vi "诊断标定3.vi"(8 "CAN端口":u16(ring), 9 "设备索引号":u16(ring), 10 "CAN卡类型":u32(ring)=21) -> ()   [LabVIEW 2013] (continued)
          tunnel: w3642 -> [w3645 w3652]
          tunnel: [w3646 w3651] -> w3641
          tunnel: [w3645 w3650] -> w3640
          frame False {
          }
          frame True {
            n2857 = global read "EV05全局变量1.vi" "授权功能"() -> (w3648:bool)
            n2858 = case shown="假" w3648 {
              tunnel: [TRUE ("发送成功") w3672] -> w3649
              frame False {
              }
              frame True {
                n2859 = local read "设备索引号"() -> (w3667:u16)
                n2860 = local read "CAN卡类型"() -> (w3668:u32)
                n2861 = local read "CAN端口"() -> (w3666:u16)
                n2862 = call "标定授权发送.vi"("CAN卡类型"=w3668, "解锁类型"=enum16{"读取", "写", "下载"}."读取", "设备索引号"=w3667, "CAN端口"=w3666, "是否连接"=TRUE, "板选择"=0, "FUNC"=u32 0) -> ("发送成功"=w3672:bool)  [unwired: 8 out]
              }
            }
            n2863 = stacked-sequence {
              tunnel: [w3656] -> w3647
              frame #0 {
                w3656 = TRUE ("控制1")
                w3660 = FALSE ("写?")
                n2864 = call <vilib>:"Set Busy.vi"("disable click? (T)"=FALSE) -> ()  [unwired: 3 in, 8 out]
                n2865 = local write "写?"(w3660) -> ()
                n2866 = global write "EV05全局变量1.vi" "写入超时"(w3660) -> ()
                n2867 = local write "平台软件版本号"(" " ("平台软件版本号")) -> ()
                n2868 = local write "控制1"(w3656) -> ()
                n2869 = local write "消除"(TRUE ("消除")) -> ()
                n2870 = property on="保存版本信息" class="Bool (严格)"("Visible"=TRUE ("可见")) -> ()  [unwired: 2 in, 2 out]
                n2871 = global write "EV05全局变量1.vi" "流控帧 2"(TRUE ("流控帧 2")) -> ()
                n2872 = local write "主从选择"(enum32{"主板", "从板"}."主板" ("主从选择")) -> ()
                n2873 = local write "清BUFF"(FALSE ("清BUFF")) -> ()
                n2874 = global write "EV05全局变量1.vi" "流控帧"(FALSE ("流控帧")) -> ()
              }
            }
            n2875 = case shown="真" w3649 {
              tunnel: w3653 -> [w3674 w3679]
              tunnel: w3652 -> [w3673 w3678]
              tunnel: [w3674 w3676] -> w3651
              tunnel: [w3673 w3675] -> w3650
              tunnel: w3647 -> [_ _]
              frame False {
              }
              frame True {
                n2876 = Enqueue Element(queue=w3679, element="平台软件版本读取" ("元素"), error in (no error)=w3678) -> (queue out=w3676:refnum<queue>, error out=w3675:errorcluster)  [unwired: 2 out]
              }
            }
          }
        }
      }
      event "模块版本读取": Value Change {
        n2877 = event-data() -> ("NewVal"=w3684:bool)  [unwired: 5 out]
        n2878 = case shown="真" w3684 {
          tunnel: w3683 -> [w3686 w3693]
          tunnel: w3682 -> [w3685 w3692]
          tunnel: [w3686 w3691] -> w3681
          tunnel: [w3685 w3690] -> w3680
          frame False {
          }
          frame True {
            n2879 = global read "EV05全局变量1.vi" "授权功能"() -> (w3688:bool)
            n2880 = case shown="假" w3688 {
              tunnel: [TRUE ("发送成功") w3711] -> w3689
              frame False {
              }
              frame True {
                n2881 = local read "设备索引号"() -> (w3706:u16)
                n2882 = local read "CAN卡类型"() -> (w3707:u32)
                n2883 = local read "CAN端口"() -> (w3705:u16)
                n2884 = call "标定授权发送.vi"("CAN卡类型"=w3707, "解锁类型"=enum16{"读取", "写", "下载"}."读取", "设备索引号"=w3706, "CAN端口"=w3705, "是否连接"=TRUE, "板选择"=0, "FUNC"=u32 0) -> ("发送成功"=w3711:bool)  [unwired: 8 out]
              }
            }
            n2885 = stacked-sequence {
              tunnel: [w3696] -> w3687
              frame #0 {
                w3696 = TRUE ("控制1")
                w3699 = FALSE ("写?")
                n2886 = call <vilib>:"Set Busy.vi"("disable click? (T)"=FALSE) -> ()  [unwired: 3 in, 8 out]
                n2887 = local write "写?"(w3699) -> ()
                n2888 = global write "EV05全局变量1.vi" "写入超时"(w3699) -> ()
                n2889 = local write "主从选择"(enum32{"主板", "从板"}."主板" ("主从选择")) -> ()
                n2890 = local write "清BUFF"(FALSE ("清BUFF")) -> ()
                n2891 = property on="保存版本信息" class="Bool (严格)"("Visible"=TRUE ("可见")) -> ()  [unwired: 2 in, 2 out]
                n2892 = global write "EV05全局变量1.vi" "流控帧 2"(TRUE ("流控帧 2")) -> ()
                n2893 = local write "控制1"(w3696) -> ()
                n2894 = local write "消除"(TRUE ("消除")) -> ()
                n2895 = global write "EV05全局变量1.vi" "流控帧"(FALSE ("流控帧")) -> ()
              }
            }
            n2896 = case shown="真" w3689 {
              tunnel: w3693 -> [w3713 w3718]
              tunnel: w3692 -> [w3712 w3717]
              tunnel: [w3713 w3715] -> w3691
              tunnel: [w3712 w3714] -> w3690
              tunnel: w3687 -> [_ _]
              frame False {
              }
              frame True {
                n2897 = Enqueue Element(queue=w3718, element="模块软件版本读取" ("元素"), error in (no error)=w3717) -> (queue out=w3715:refnum<queue>, error out=w3714:errorcluster)  [unwired: 2 out]
              }
            }
          }
        }
      }
      event "保存版本信息": Value Change {
        n2898 = event-data() -> ("NewVal"=w3719:bool)  [unwired: 6 out]
        n2899 = case shown="真" w3719 {
          frame False {
          }
          frame True {
            n2900 = stacked-sequence {
              seq-local: [w3723 _] -> [_ w3725]
              seq-local: [w3722 _] -> [_ w3724]
              frame #0 {
                n2901 = call "请输入从板个数"() -> ("从板个数"=w3723:dbl, "确定"=w3722:bool)  [unwired: 17 in, 1 out]
              }
              frame #1 {
                n2902 = case shown="真" w3724 {
                  tunnel: w3725 -> [_ w3728]
                  frame False {
                  }
                  frame True {
                    n2903 = call <vilib>:"Application Directory.vi"() -> ("Application Directory"=w3740:path)
                    n2904 = Build Path(base path=w3740, name or relative path="SaveData" ("名称或相对路径")) -> (appended path=w3738:path)
                    n2905 = local read "模块版本名称"() -> (w3733:string[][])
                    n2906 = local read "项目软件版本"() -> (w3730:string[])
                    n2907 = local read "模块版本值"() -> (w3732:string[][])
                    n2908 = local read "平台软件版本"() -> (w3729:string[])
                    n2909 = local read "模块个数"() -> (w3726:u8[])
                    n2910 = local read "硬件版本"() -> (w3731:string[])
                    n2911 = call "文件对话框3"("start path"=w3738, "prompt"="选择要保存数据的位置", "default name"="BMS版本信息.txt") -> ("selected path"=w3734:path, "cancelled"=w3735:bool)  [unwired: 9 in, 2 out]
                    n2912 = Increment(x=w3728) -> (x+1=w3727:dbl)
                    n2913 = for {
                      N: w3727 -> [_]
                      tunnel: w3735 -> [w3756]
                      tunnel: w3734 -> [w3755]
                      tunnel: w3733 -> [w3745] mode=indexing
                      tunnel: w3732 -> [w3743] mode=indexing
                      tunnel: w3731 -> [w3750] mode=indexing
                      tunnel: w3730 -> [w3749] mode=indexing
                      tunnel: w3729 -> [w3748] mode=indexing
                      tunnel: w3726 -> [w3741] mode=indexing
                      i -> [w3747]
                      w3753 = ""
                      w3760 = 0 ("索引")
                      n2914 = case shown="0, 默认" w3747 {
                        selector: w3747 -> [_ w3774]
                        tunnel: ["主板版本信息" w3775] -> w3765
                        tunnel: [FALSE TRUE] -> w3751
                        frame 0, Default {
                        }
                        frame 1.. {
                          n2915 = Number To Decimal String(number=w3774) -> (decimal integer string=w3773:string)  [unwired: 1 in]
                          n2916 = Concatenate Strings("从板", w3773, "版本信息") -> (w3775:string)
                        }
                      }
                      n2917 = Increment(x=w3741) -> (x+1=w3742:u8)
                      n2918 = Array Subset(array=w3745, length=w3742) -> (w3746:string[])  [unwired: 1 in]
                      n2919 = Array Subset(array=w3743, length=w3742) -> (w3744:string[])  [unwired: 1 in]
                      n2920 = Build Array(w3753, w3748, w3749, w3750, w3753) -> (w3759:string[])
                      n2921 = Build Array(w3765, "平台软件版本号", "项目软件版本号", "硬件版本号", "模块版本号") -> (w3761:string[])
                      n2922 = Insert Into Array(array=w3746, index=w3760, new element=w3761) -> (w3758:string[])
                      n2923 = Insert Into Array(array=w3744, index=w3760, new element=w3759) -> (w3757:string[])
                      n2924 = Build Array(w3758, w3757) -> (w3754:string[][])
                      n2925 = case shown="假" w3756 {
                        tunnel: w3755 -> [w3769 _]
                        tunnel: w3754 -> [w3768 _]
                        tunnel: w3751 -> [w3766 _]
                        frame False {
                          n2926 = call-poly <vilib>:"Write To Spreadsheet File.vi"("transpose? (no:F)"=TRUE, "append to file? (new file:F)"=w3766, "2D data"=w3768, "file path (dialog if empty)"=w3769) -> ()  [unwired: 4 in, 1 out]
                        }
                        frame True {
                        }
                      }
                    }
                  }
                }
              }
            }
          }
        }
      }
      event "单个写入": Value Change {
        n2927 = event-data() -> ("NewVal"=w3782:bool)  [unwired: 5 out]
        n2928 = case shown="真" w3782 {
          tunnel: w3781 -> [w3784 w3791]
          tunnel: w3780 -> [w3783 w3790]
          tunnel: [w3784 w3789] -> w3779
          tunnel: [w3783 w3788] -> w3778
          frame False {
          }
          frame True {
            w3786 = FALSE ("流控帧")
            w3785 = TRUE ("流控帧 2")
            n2929 = disable-structure shown="禁用" {
              disable-tunnel: [w3800 TRUE ("发送成功")] -> w3787
              frame Disabled {
                n2930 = local read "主从选择"() -> (w3792:enum32{"主板", "从板"})
                n2931 = case shown="\"主板\", 默认" w3792 {
                  tunnel: [0.0 ("FUNC") w3802] -> w3797
                  frame "主板", Default {
                  }
                  frame "从板" {
                    n2932 = local read "从板号"() -> (w3802:u8)
                  }
                }
                n2933 = local read "设备索引号"() -> (w3794:u16)
                n2934 = local read "CAN卡类型"() -> (w3795:u32)
                n2935 = local read "CAN端口"() -> (w3793:u16)
                n2936 = call "标定授权发送.vi"("CAN卡类型"=w3795, "解锁类型"=enum16{"读取", "写", "下载"}."写", "设备索引号"=w3794, "CAN端口"=w3793, "是否连接"=TRUE, "板选择"=0, "FUNC"=w3797) -> ("发送成功"=w3800:bool)  [unwired: 8 out]
              }
              frame Enabled {
              }
            }
            n2937 = case shown="真" w3787 {
              tunnel: w3791 -> [w3805 w3809]
              tunnel: w3790 -> [w3804 w3808]
              tunnel: [w3805 w3811] -> w3789
              tunnel: [w3804 w3810] -> w3788
              frame False {
              }
              frame True {
                n2938 = Flush Queue(queue=w3809, error in (no error)=w3808) -> (queue out=w3807:refnum<queue>, error out=w3806:errorcluster)  [unwired: 1 out]
                n2939 = Enqueue Element(queue=w3807, element="单个写入" ("元素"), error in (no error)=w3806) -> (queue out=w3811:refnum<queue>, error out=w3810:errorcluster)  [unwired: 2 out]
              }
            }
            n2940 = global write "EV05全局变量1.vi" "读取超时"(w3786) -> ()
            n2941 = global write "EV05全局变量1.vi" "流控帧"(w3786) -> ()
            n2942 = local write "消除"(w3785) -> ()
            n2943 = local write "控制1"(w3785) -> ()
            n2944 = global write "EV05全局变量1.vi" "流控帧 2"(w3785) -> ()
            n2945 = local write "写?"(w3785) -> ()
          }
        }
      }
      event "全部写入": Value Change {
        n2946 = event-data() -> ("NewVal"=w3817:bool)  [unwired: 5 out]
        n2947 = case shown="真" w3817 {
          tunnel: w3816 -> [w3819 w3827]
          tunnel: w3815 -> [w3818 w3826]
          tunnel: [w3819 w3825] -> w3814
          tunnel: [w3818 w3824] -> w3813
          frame False {
          }
          frame True {
            w3821 = FALSE ("流控帧")
            w3820 = TRUE ("流控帧 2")
            n2948 = global read "EV05全局变量1.vi" "授权功能"() -> (w3822:bool)
            n2949 = case shown="真" w3822 {
              tunnel: [TRUE ("发送成功") w3837] -> w3823
              frame False {
              }
              frame True {
                n2950 = local read "主从选择"() -> (w3829:enum32{"主板", "从板"})
                n2951 = case shown="\"从板\"" w3829 {
                  tunnel: [0.0 ("FUNC") w3839] -> w3830
                  frame "主板", Default {
                  }
                  frame "从板" {
                    n2952 = local read "从板号"() -> (w3839:u8)
                  }
                }
                n2953 = local read "设备索引号"() -> (w3832:u16)
                n2954 = local read "CAN卡类型"() -> (w3833:u32)
                n2955 = local read "CAN端口"() -> (w3831:u16)
                n2956 = call "标定授权发送.vi"("CAN卡类型"=w3833, "解锁类型"=enum16{"读取", "写", "下载"}."写", "设备索引号"=w3832, "CAN端口"=w3831, "是否连接"=TRUE, "板选择"=0, "FUNC"=w3830) -> ("发送成功"=w3837:bool)  [unwired: 8 out]
              }
            }
            n2957 = case shown="真" w3823 {
              tunnel: w3827 -> [w3841 w3845]
              tunnel: w3826 -> [w3840 w3844]
              tunnel: [w3841 w3847] -> w3825
              tunnel: [w3840 w3846] -> w3824
              frame False {
              }
              frame True {
                n2958 = Flush Queue(queue=w3845, error in (no error)=w3844) -> (queue out=w3843:refnum<queue>, error out=w3842:errorcluster)  [unwired: 1 out]
                n2959 = Enqueue Element(queue=w3843, element="全部写入" ("元素"), error in (no error)=w3842) -> (queue out=w3847:refnum<queue>, error out=w3846:errorcluster)  [unwired: 1 in, 1 out]
              }
            }
            n2960 = global write "EV05全局变量1.vi" "读取超时"(w3821) -> ()
            n2961 = global write "EV05全局变量1.vi" "流控帧"(w3821) -> ()
            n2962 = local write "消除"(w3820) -> ()
            n2963 = local write "控制1"(w3820) -> ()
            n2964 = global write "EV05全局变量1.vi" "流控帧 2"(w3820) -> ()
            n2965 = local write "写?"(w3820) -> ()
          }
        }
      }
      event "单个读取": Value Change {
        n2966 = event-data() -> ("NewVal"=w3853:bool)  [unwired: 5 out]
        n2967 = case shown="真" w3853 {
          tunnel: w3852 -> [w3855 w3863]
          tunnel: w3851 -> [w3854 w3862]
          tunnel: [w3855 w3861] -> w3850
          tunnel: [w3854 w3860] -> w3849
          frame False {
          }
          frame True {
            w3856 = FALSE ("流控帧")
            w3857 = TRUE ("流控帧 2")
            n2968 = global read "EV05全局变量1.vi" "授权功能"() -> (w3858:bool)
            n2969 = case shown="假" w3858 {
              tunnel: [TRUE ("发送成功") w3872] -> w3859
              frame False {
              }
              frame True {
                n2970 = local read "设备索引号"() -> (w3866:u16)
                n2971 = local read "CAN卡类型"() -> (w3867:u32)
                n2972 = local read "CAN端口"() -> (w3865:u16)
                n2973 = call "标定授权发送.vi"("CAN卡类型"=w3867, "解锁类型"=enum16{"读取", "写", "下载"}."读取", "设备索引号"=w3866, "CAN端口"=w3865, "是否连接"=TRUE, "板选择"=0, "FUNC"=u32 1) -> ("发送成功"=w3872:bool)  [unwired: 8 out]
              }
            }
            n2974 = case shown="真" w3859 {
              tunnel: w3863 -> [w3874 w3878]
              tunnel: w3862 -> [w3873 w3876]
              tunnel: [w3874 w3880] -> w3861
              tunnel: [w3873 w3879] -> w3860
              frame False {
              }
              frame True {
                n2975 = Flush Queue(queue=w3878, error in (no error)=w3876) -> (queue out=w3877:refnum<queue>, error out=w3875:errorcluster)  [unwired: 1 out]
                n2976 = Enqueue Element(queue=w3877, element="单个读取" ("元素"), error in (no error)=w3875) -> (queue out=w3880:refnum<queue>, error out=w3879:errorcluster)  [unwired: 2 out]
              }
            }
            n2977 = global write "EV05全局变量1.vi" "写入超时"(w3856) -> ()
            n2978 = global write "EV05全局变量1.vi" "流控帧"(w3856) -> ()
            n2979 = local write "写?"(w3856) -> ()
            n2980 = local write "消除"(w3857) -> ()
            n2981 = local write "控制1"(w3857) -> ()
            n2982 = global write "EV05全局变量1.vi" "流控帧 2"(w3857) -> ()
          }
        }
      }
      event "全部读取": Value Change {
        n2983 = event-data() -> ("NewVal"=w3886:bool)  [unwired: 5 out]
        n2984 = case shown="真" w3886 {
          tunnel: w3885 -> [w3888 w3892]
          tunnel: w3884 -> [w3887 w3891]
          tunnel: [w3888 w3890] -> w3883
          tunnel: [w3887 w3889] -> w3882
          frame False {
          }
          frame True {
            n2985 = stacked-sequence {
              seq-local: [w3897 _] -> [_ _]
              seq-local: [w3896 _] -> [_ _]
              tunnel: w3892 -> [w3899 w3929]
              tunnel: w3891 -> [w3898 w3928]
              tunnel: [_ w3933] -> w3890
              tunnel: [_ w3932] -> w3889
              frame #0 {
                w3893 = FALSE ("布尔")
                n2986 = local read "路径"() -> (w3895:path)
                n2987 = Empty String/Path?(string/path=w3895) -> (empty?=w3894:bool)
                n2988 = case shown="假" w3894 {
                  tunnel: w3899 -> [w3907 w3925]
                  tunnel: w3898 -> [w3906 w3924]
                  tunnel: [w3903 w3924] -> w3897
                  tunnel: [w3902 w3925] -> w3896
                  frame False {
                    n2989 = global read "EV05全局变量1.vi" "授权功能"() -> (w3904:bool)
                    n2990 = case shown="真" w3904 {
                      tunnel: [TRUE ("发送成功") w3916] -> w3905
                      frame False {
                      }
                      frame True {
                        n2991 = local read "设备索引号"() -> (w3910:u16)
                        n2992 = local read "CAN卡类型"() -> (w3911:u32)
                        n2993 = local read "CAN端口"() -> (w3909:u16)
                        n2994 = call "标定授权发送.vi"("CAN卡类型"=w3911, "解锁类型"=enum16{"读取", "写", "下载"}."读取", "设备索引号"=w3910, "CAN端口"=w3909, "是否连接"=TRUE, "板选择"=0, "FUNC"=u32 1) -> ("发送成功"=w3916:bool)  [unwired: 8 out]
                      }
                    }
                    n2995 = case shown="真" w3905 {
                      tunnel: w3907 -> [w3918 w3923]
                      tunnel: w3906 -> [w3917 w3922]
                      tunnel: [w3918 w3920] -> w3902
                      tunnel: [w3917 w3919] -> w3903
                      frame False {
                      }
                      frame True {
                        n2996 = Enqueue Element(queue=w3923, element="读配置文件" ("元素"), error in (no error)=w3922) -> (queue out=w3920:refnum<queue>, error out=w3919:errorcluster)  [unwired: 2 out]
                      }
                    }
                    n2997 = local write "布尔"(FALSE ("布尔")) -> ()
                    n2998 = Wait Until Next ms Multiple(millisecond multiple=u32 200 ("毫秒倍数")) -> ()  [unwired: 1 out]
                  }
                  frame True {
                  }
                }
                n2999 = local write "1 6"(w3893) -> ()
                n3000 = local write "1 7"(w3893) -> ()
                n3001 = local write "1 8"(w3893) -> ()
                n3002 = local write "1 9"(w3893) -> ()
                n3003 = local write "1 10"(w3893) -> ()
                n3004 = local write "1 12"(w3893) -> ()
              }
              frame #1 {
                w3926 = FALSE ("流控帧")
                w3927 = TRUE ("流控帧 2")
                n3005 = global read "EV05全局变量1.vi" "授权功能"() -> (w3930:bool)
                n3006 = case shown="假" w3930 {
                  tunnel: [TRUE ("发送成功") w3942] -> w3931
                  frame False {
                  }
                  frame True {
                    n3007 = local read "设备索引号"() -> (w3936:u16)
                    n3008 = local read "CAN卡类型"() -> (w3937:u32)
                    n3009 = local read "CAN端口"() -> (w3935:u16)
                    n3010 = call "标定授权发送.vi"("CAN卡类型"=w3937, "解锁类型"=enum16{"读取", "写", "下载"}."读取", "设备索引号"=w3936, "CAN端口"=w3935, "是否连接"=TRUE, "板选择"=0, "FUNC"=u32 1) -> ("发送成功"=w3942:bool)  [unwired: 8 out]
                  }
                }
                n3011 = case shown="真" w3931 {
                  tunnel: w3929 -> [w3944 w3945]
                  tunnel: w3928 -> [w3943 w3948]
                  tunnel: [w3944 w3950] -> w3933
                  tunnel: [w3943 w3949] -> w3932
                  frame False {
                  }
                  frame True {
                    n3012 = Flush Queue(queue=w3945, error in (no error)=w3948) -> (queue out=w3946:refnum<queue>, error out=w3947:errorcluster)  [unwired: 1 out]
                    n3013 = Enqueue Element(queue=w3946, element="全部读取" ("元素"), error in (no error)=w3947) -> (queue out=w3950:refnum<queue>, error out=w3949:errorcluster)  [unwired: 2 out]
                  }
                }
                n3014 = global write "EV05全局变量1.vi" "写入超时"(w3926) -> ()
                n3015 = global write "EV05全局变量1.vi" "流控帧"(w3926) -> ()
                n3016 = local write "写?"(w3926) -> ()
                n3017 = local write "消除"(w3927) -> ()
                n3018 = local write "控制1"(w3927) -> ()
                n3019 = global write "EV05全局变量1.vi" "流控帧 2"(w3927) -> ()
              }
            }
          }
        }
      }
      event "开启均衡": Value Change {
        n3020 = event-data() -> ("NewVal"=w3956:bool)  [unwired: 5 out]
        n3021 = case shown="真" w3956 {
          tunnel: w3955 -> [w3958 w3965]
          tunnel: w3954 -> [w3957 w3964]
          tunnel: [w3958 w3963] -> w3953
          tunnel: [w3957 w3962] -> w3952
          frame False {
          }
          frame True {
            n3022 = global read "EV05全局变量1.vi" "授权功能"() -> (w3960:bool)
            n3023 = case shown="假" w3960 {
              tunnel: [TRUE ("发送成功") w3975] -> w3961
              frame False {
              }
              frame True {
                n3024 = local read "主从选择"() -> (w3967:enum32{"主板", "从板"})
                n3025 = case shown="\"从板\"" w3967 {
                  tunnel: [0.0 ("FUNC") w3977] -> w3968
                  frame "主板", Default {
                  }
                  frame "从板" {
                    n3026 = local read "从板号"() -> (w3977:u8)
                  }
                }
                n3027 = local read "设备索引号"() -> (w3970:u16)
                n3028 = local read "CAN卡类型"() -> (w3971:u32)
                n3029 = local read "CAN端口"() -> (w3969:u16)
                n3030 = call "标定授权发送.vi"("CAN卡类型"=w3971, "解锁类型"=enum16{"读取", "写", "下载"}."写", "设备索引号"=w3970, "CAN端口"=w3969, "是否连接"=TRUE, "板选择"=0, "FUNC"=w3968) -> ("发送成功"=w3975:bool)  [unwired: 8 out]
              }
            }
            n3031 = case shown="真" w3961 {
              tunnel: w3965 -> [w3979 w3984]
              tunnel: w3964 -> [w3978 w3983]
              tunnel: [w3979 w3981] -> w3963
              tunnel: [w3978 w3980] -> w3962
              frame False {
              }
              frame True {
                n3032 = Enqueue Element(queue=w3984, element="开启均衡" ("元素"), error in (no error)=w3983) -> (queue out=w3981:refnum<queue>, error out=w3980:errorcluster)  [unwired: 2 out]
              }
            }
            n3033 = call <vilib>:"Set Busy.vi"("disable click? (T)"=TRUE) -> ()  [unwired: 3 in, 8 out]
          }
        }
      }
      event "关闭均衡": Value Change {
        n3034 = event-data() -> ("NewVal"=w3989:bool)  [unwired: 5 out]
        n3035 = case shown="真" w3989 {
          tunnel: w3988 -> [w3991 w3998]
          tunnel: w3987 -> [w3990 w3997]
          tunnel: [w3991 w3996] -> w3986
          tunnel: [w3990 w3995] -> w3985
          frame False {
          }
          frame True {
            n3036 = global read "EV05全局变量1.vi" "授权功能"() -> (w3993:bool)
            n3037 = case shown="假" w3993 {
              tunnel: [TRUE ("发送成功") w4008] -> w3994
              frame False {
              }
              frame True {
                n3038 = local read "主从选择"() -> (w4000:enum32{"主板", "从板"})
                n3039 = case shown="\"从板\"" w4000 {
                  tunnel: [0.0 ("FUNC") w4010] -> w4001
                  frame "主板", Default {
                  }
                  frame "从板" {
                    n3040 = local read "从板号"() -> (w4010:u8)
                  }
                }
                n3041 = local read "设备索引号"() -> (w4003:u16)
                n3042 = local read "CAN卡类型"() -> (w4004:u32)
                n3043 = local read "CAN端口"() -> (w4002:u16)
                n3044 = call "标定授权发送.vi"("CAN卡类型"=w4004, "解锁类型"=enum16{"读取", "写", "下载"}."写", "设备索引号"=w4003, "CAN端口"=w4002, "是否连接"=TRUE, "板选择"=0, "FUNC"=w4001) -> ("发送成功"=w4008:bool)  [unwired: 8 out]
              }
            }
            n3045 = case shown="真" w3994 {
              tunnel: w3998 -> [w4012 w4017]
              tunnel: w3997 -> [w4011 w4016]
              tunnel: [w4012 w4014] -> w3996
              tunnel: [w4011 w4013] -> w3995
              frame False {
              }
              frame True {
                n3046 = Enqueue Element(queue=w4017, element="关闭均衡" ("元素"), error in (no error)=w4016) -> (queue out=w4014:refnum<queue>, error out=w4013:errorcluster)  [unwired: 2 out]
              }
            }
            n3047 = call <vilib>:"Set Busy.vi"("disable click? (T)"=TRUE) -> ()  [unwired: 3 in, 8 out]
          }
        }
      }
      event "强制开启均衡": Value Change {
        n3048 = event-data() -> ("NewVal"=w4022:bool)  [unwired: 5 out]
        n3049 = case shown="真" w4022 {
          tunnel: w4021 -> [w4024 w4031]
          tunnel: w4020 -> [w4023 w4030]
          tunnel: [w4024 w4029] -> w4019
          tunnel: [w4023 w4028] -> w4018
          frame False {
          }
          frame True {
            n3050 = global read "EV05全局变量1.vi" "授权功能"() -> (w4026:bool)
            n3051 = case shown="假" w4026 {
              tunnel: [TRUE ("发送成功") w4041] -> w4027
              frame False {
              }
              frame True {
                n3052 = local read "主从选择"() -> (w4033:enum32{"主板", "从板"})
                n3053 = case shown="\"从板\"" w4033 {
                  tunnel: [0.0 ("FUNC") w4043] -> w4034
                  frame "主板", Default {
                  }
                  frame "从板" {
                    n3054 = local read "从板号"() -> (w4043:u8)
                  }
                }
                n3055 = local read "设备索引号"() -> (w4036:u16)
                n3056 = local read "CAN卡类型"() -> (w4037:u32)
                n3057 = local read "CAN端口"() -> (w4035:u16)
                n3058 = call "标定授权发送.vi"("CAN卡类型"=w4037, "解锁类型"=enum16{"读取", "写", "下载"}."写", "设备索引号"=w4036, "CAN端口"=w4035, "是否连接"=TRUE, "板选择"=0, "FUNC"=w4034) -> ("发送成功"=w4041:bool)  [unwired: 8 out]
              }
            }
            n3059 = case shown="真" w4027 {
              tunnel: w4031 -> [w4045 w4050]
              tunnel: w4030 -> [w4044 w4049]
              tunnel: [w4045 w4047] -> w4029
              tunnel: [w4044 w4046] -> w4028
              frame False {
              }
              frame True {
                n3060 = Enqueue Element(queue=w4050, element="强制均衡" ("元素"), error in (no error)=w4049) -> (queue out=w4047:refnum<queue>, error out=w4046:errorcluster)  [unwired: 2 out]
              }
            }
            n3061 = call <vilib>:"Set Busy.vi"("disable click? (T)"=TRUE) -> ()  [unwired: 3 in, 8 out]
          }
        }
      }
    }
    n3062 = Unbundle By Name(w1237) -> ("status"=w1236:bool)
    n3063 = Or(x=w1236, y=w1238) -> (x .or. y?=w1239:bool)
  }
  n3064 = while {
    tunnel: w36 -> [w4056]
    tunnel: w35 -> [w4055]
    stop <- w4052 stop-if-true
    n3065 = local read "停止"() -> (w4052:bool)
    n3066 = Dequeue Element(queue=w4056, timeout in ms (-1)=100 ("超时毫秒(-1)"), error in (no error)=w4055) -> (element=w4054:string, error out=w4053:errorcluster)  [unwired: 2 out]
    n3067 = case shown="无错误" w4053 {
      tunnel: w4054 -> [w4057 _]
      frame No Error {
        n3068 = case shown="\"读配置文件\"" w4057 {
          frame "假", Default {
            n3069 = local write "强制终止读写标记"(FALSE ("强制终止读写标记")) -> ()
          }
          frame "单个写入" {
            n3070 = local read "主从选择"() -> (w4067:enum32{"主板", "从板"})
            n3071 = case shown="\"从板\"" w4067 {
              tunnel: [w4078 w4093] -> w4064
              tunnel: [0.0 w4091] -> w4068
              tunnel: [_ w4092] -> w4066
              tunnel: [w4076 _] -> w4065
              frame "主板", Default {
                n3072 = flat-sequence {
                  tunnel: [w4090] -> w4076
                  frame #0 {
                    n3073 = control-ref of="高压参数"() -> (w4081:refnum<vi>)
                    n3074 = control-ref of="电池信息"() -> (w4082:refnum<vi>)
                    n3075 = control-ref of="一级故障"() -> (w4088:refnum<vi>)
                    n3076 = control-ref of="一级故障 2"() -> (w4086:refnum<vi>)
                    n3077 = control-ref of="一级故障 3"() -> (w4085:refnum<vi>)
                    n3078 = control-ref of="加热控制参数"() -> (w4084:refnum<vi>)
                    n3079 = control-ref of="充电控制参数"() -> (w4083:refnum<vi>)
                    n3080 = control-ref of="项目信息"() -> (w4087:refnum<vi>)
                    n3081 = control-ref of="项目信息2"() -> (w4089:refnum<vi>)
                    n3082 = local read "主板数据"() -> (w4079:T4)
                    n3083 = Bundle(cluster=w4079, "项目信息"=w4087, "一级故障 4"=w4089, "一级故障"=w4088, "一级故障 2"=w4086, "一级故障 3"=w4085, "加热控制参数"=w4084, "充电控制参数"=w4083, "高压参数"=w4081, "电池信息"=w4082) -> (w4080:T4)
                    n3084 = local write "主板数据"(w4080) -> ()
                  }
                  frame #1 {
                    n3085 = control-ref of="主板数据"() -> (w4090:refnum<vi>)
                  }
                }
                n3086 = local read "主板选项"() -> (w4078:string)
              }
              frame "从板" {
                n3087 = stacked-sequence {
                  tunnel: [_ w4104] -> w4092
                  frame #0 {
                    n3088 = control-ref of="从板号"() -> (w4103:refnum<vi>)
                    n3089 = control-ref of="项目信息 2"() -> (w4102:refnum<vi>)
                    n3090 = control-ref of="均衡参数"() -> (w4097:refnum<vi>)
                    n3091 = control-ref of="加热控制参数"() -> (w4101:refnum<vi>)
                    n3092 = control-ref of="一级故障(从板)"() -> (w4100:refnum<vi>)
                    n3093 = control-ref of="二级故障(从板)"() -> (w4099:refnum<vi>)
                    n3094 = control-ref of="三级故障(从板)"() -> (w4098:refnum<vi>)
                    n3095 = control-ref of="电池组信息"() -> (w4094:refnum<vi>)
                    n3096 = local read "从板信息"() -> (w4095:T2)
                    n3097 = Bundle(cluster=w4095, "从板号"=w4103, "项目信息 2"=w4102, "加热控制参数"=w4101, "一级故障(从板)"=w4100, "二级故障(从板)"=w4099, "三级故障(从板)"=w4098, "电池组信息(从板)"=w4094, "均衡参数"=w4097) -> (w4096:T2)
                    n3098 = local write "从板信息"(w4096) -> ()
                  }
                  frame #1 {
                    n3099 = control-ref of="从板信息"() -> (w4104:refnum<vi>)
                  }
                }
                n3100 = local read "从板选项"() -> (w4093:string)
                n3101 = local read "从板号"() -> (w4091:u8)
              }
            }
            n3102 = local read "从板个数"() -> (w4069:dbl)
            n3103 = local read "二维码信息 2"() -> (w4059:string)
            n3104 = local read "二维码信息"() -> (w4060:string)
            n3105 = local read "快换"() -> (w4070:bool)
            n3106 = call "输入数据解析.vi"("单个参数补充"=w4069, "从板号"=w4068, "主板二维码"=w4060, "从板二维码"=w4059, "主板引用"=w4065, "从板引用"=w4066, "主板选项"=w4064, "枚举"=w4067, "快换"=w4070) -> ("输出数组"=w4074:dbl[][], "数组长度"=w4073:dbl[], "循环次数"=w4063:i32, "命令"=w4072:u32, "名称"=w4062:string[], "命令序号"=w4071:u32[])  [unwired: 1 out]
            n3107 = for {
              N: w4063 -> [w4110]
              tunnel: w4074 -> [w4120]
              tunnel: w4073 -> [w4119]
              tunnel: w4072 -> [w4118]
              tunnel: w4071 -> [w4117]
              tunnel: w4068 -> [w4108]
              tunnel: w4064 -> [w4116]
              tunnel: w4062 -> [w4112]
              tunnel: [w4105] -> w4061
              i -> [w4111]
              n3108 = Index Array(array=w4120, index (row)=w4111) -> (element=w4115:dbl[])  [unwired: 1 in]
              n3109 = Index Array(array=w4119, index=w4111) -> (element=w4114:dbl)
              n3110 = Index Array(array=w4112, index=w4111) -> (element=w4109:string)
              n3111 = case shown="\"假\", 默认" w4109 {
                tunnel: [w4122 w4123] -> w4107
                tunnel: w4108 -> [w4122 _]
                tunnel: [TRUE ("确定") w4124] -> w4106
                frame "假", Default {
                }
                frame "从板号" {
                  n3112 = call "请输入当前从板板号"() -> ("当前从板板号"=w4123:dbl, "确定"=w4124:bool)  [unwired: 17 in, 1 out]
                  n3113 = local write "当前从板板号"(w4123) -> ()
                }
              }
              n3114 = Index Array(array=w4117, index=w4111) -> (element=w4113:u32)
              n3115 = global write "全局 1.vi" "名称"(w4109) -> ()
              n3116 = case shown="真" w4106 {
                tunnel: w4118 -> [_ w4134]
                tunnel: w4116 -> [_ w4133]
                tunnel: w4115 -> [_ w4132]
                tunnel: w4114 -> [_ w4131]
                tunnel: w4113 -> [_ w4130]
                tunnel: w4111 -> [_ w4129]
                tunnel: w4109 -> [_ w4128]
                tunnel: w4110 -> [_ w4127]
                tunnel: w4107 -> [_ w4126]
                tunnel: [_ w4125] -> w4105
                frame False {
                  n3117 = call <vilib>:"Unset Busy.vi"() -> ()  [unwired: 11 in, 1 out]
                }
                frame True {
                  n3118 = stacked-sequence {
                    seq-local: [_ _ _ w4162 _ _] -> [_ _ _ _ w4171 _]
                    tunnel: w4132 -> [_ _ w4147 _ _ _]
                    tunnel: w4131 -> [_ _ w4146 _ _ _]
                    tunnel: w4134 -> [_ _ w4140 _ _ _]
                    tunnel: w4130 -> [_ _ w4138 _ _ _]
                    tunnel: w4133 -> [_ _ _ _ _ _]
                    tunnel: w4129 -> [_ _ _ _ _ w4182]
                    tunnel: w4128 -> [_ _ _ _ w4170 _]
                    tunnel: w4127 -> [_ _ _ _ _ w4183]
                    tunnel: w4126 -> [_ _ w4139 _ _ _]
                    tunnel: [_ _ _ _ _ w4180] -> w4125
                    frame #0 {
                      w4136 = FALSE ("流控帧")
                      w4135 = TRUE ("流控帧 2")
                      n3119 = call <vilib>:"Set Busy.vi"("disable click? (T)"=w4136) -> ()  [unwired: 3 in, 8 out]
                      n3120 = global write "EV05全局变量1.vi" "读取超时"(w4136) -> ()
                      n3121 = global write "EV05全局变量1.vi" "流控帧"(w4136) -> ()
                      n3122 = local write "消除"(w4135) -> ()
                      n3123 = local write "控制1"(w4135) -> ()
                      n3124 = global write "EV05全局变量1.vi" "流控帧 2"(w4135) -> ()
                      n3125 = local write "写?"(w4135) -> ()
                    }
                    frame #1 {
                      n3126 = Wait Until Next ms Multiple(millisecond multiple=u32 50 ("毫秒倍数")) -> ()  [unwired: 1 out]
                    }
                    frame #2 {
                      n3127 = local read "设备索引号"() -> (w4142:u16)
                      n3128 = local read "CAN卡类型"() -> (w4143:u32)
                      n3129 = Increment(x=w4146) -> (x+1=w4145:dbl)
                      n3130 = local read "CAN端口"() -> (w4141:u16)
                      n3131 = local write "命令"(w4140) -> ()
                      n3132 = local write "命令序号"(w4138) -> ()
                      n3133 = Reshape Array(w4147, w4145) -> (w4144:dbl[])
                      n3134 = stacked-sequence {
                        tunnel: w4144 -> [_ w4161]
                        tunnel: w4143 -> [w4150 w4160]
                        tunnel: w4142 -> [w4149 w4159]
                        tunnel: w4141 -> [w4148 w4158]
                        tunnel: w4140 -> [_ w4157]
                        tunnel: w4139 -> [_ w4156]
                        tunnel: w4138 -> [_ w4155]
                        frame #0 {
                          n3135 = disable-structure shown="禁用" {
                            disable-tunnel: w4150 -> [w4153 _]
                            disable-tunnel: w4149 -> [w4152 _]
                            disable-tunnel: w4148 -> [w4151 _]
                            frame Disabled {
                              n3136 = dll-call lib="PTH1tabs FBluewave New EnergySVN_Work\nBNET01_BMStrunkBMS_Monitor_增加二维码data\nkerneldlls\nusbcan.dll" fn="VCI_ClearBuffer"("DeviceType"=w4153, "DeviceInd"=w4152, "CANInd"=w4151) -> (error out=w4154:errorcluster)  [unwired: 4 in, 4 out]
                              n3137 = call <vilib>:"Clear Errors.vi"("error in (no error)"=w4154) -> ()  [unwired: 6 in, 1 out]
                            }
                            frame Enabled {
                            }
                          }
                        }
                        frame #1 {
                          n3138 = call "多帧发送机制(EV05).vi"("can卡类型"=w4160, "设备索引号"=w4159, "CAN端口"=w4158, "命令"=w4157, "板号"=w4156, "命令序号"=w4155, "输入数据"=w4161) -> ()  [unwired: 1 in, 12 out]
                        }
                      }
                    }
                    frame #3 {
                      n3139 = while {
                        tunnel: [w4164] -> w4162
                        i -> [w4168]
                        stop <- w4165 stop-if-true
                        n3140 = local read "强制终止读写标记"() -> (w4163:bool)
                        n3141 = global read "EV05全局变量1.vi" "读取超时"() -> (w4164:bool)
                        n3142 = Greater Or Equal?(x=w4168, y=30) -> (x >= y?=w4166:bool)
                        n3143 = Wait Until Next ms Multiple(millisecond multiple=u32 100 ("毫秒倍数")) -> ()  [unwired: 1 out]
                        n3144 = Compound Arithmetic op=OR(w4163, w4164, w4166) -> (w4165:bool)
                      }
                    }
                    frame #4 {
                      n3145 = case shown="假" w4171 {
                        tunnel: w4170 -> [w4172 w4178]
                        frame False {
                          n3146 = control-ref of="结果"() -> (w4176:refnum<vi>)
                          n3147 = Concatenate Strings(w4172, "       写入失败" ("字符串")) -> (w4175:string)
                          n3148 = Build Array(w4175) -> (w4174:string[])
                          n3149 = call "表格编辑.vi"("新元素/子数组"=w4174, "活动单元格:单元格背景色"=u32 16740749, "MCListbox引用句柄"=w4176) -> ()  [unwired: 9 out]
                        }
                        frame True {
                          n3150 = case shown="\"从板号\"" w4178 {
                            frame "假", Default {
                            }
                            frame "从板号" {
                              n3151 = local read "从板号"() -> (w4179:u8)
                              n3152 = local write "当前从板板号"(w4179) -> ()
                            }
                          }
                        }
                      }
                      n3153 = call <vilib>:"Unset Busy.vi"() -> ()  [unwired: 2 in, 10 out]
                    }
                    frame #5 {
                      n3154 = Increment(x=w4182) -> (x+1=w4181:i32)
                      n3155 = Equal?(x=w4183, y=w4181) -> (x = y?=w4180:bool)
                      n3156 = case shown="真" w4180 {
                        frame False {
                        }
                        frame True {
                          n3157 = control-ref of="结果"() -> (w4187:refnum<vi>)
                          n3158 = Concatenate Strings("写入完成" ("字符串")) -> (w4186:string)
                          n3159 = Build Array(w4186) -> (w4185:string[])
                          n3160 = call "表格编辑.vi"("新元素/子数组"=w4185, "活动单元格:单元格背景色"=u32 21937, "MCListbox引用句柄"=w4187) -> ()  [unwired: 9 out]
                        }
                      }
                    }
                  }
                }
              }
            }
            n3161 = stacked-sequence {
              tunnel: w4061 -> [_]
              frame #0 {
                n3162 = call <vilib>:"Unset Busy.vi"() -> ()  [unwired: 2 in, 10 out]
                n3163 = local write "强制终止读写标记"(FALSE ("强制停止")) -> ()
              }
            }
          }
          frame "全部写入" {
            n3164 = local read "主从选择"() -> (w4194:enum32{"主板", "从板"})
            n3165 = case shown="\"主板\", 默认" w4194 {
              tunnel: [string[] ["项目信息", "一级故障阀值", "二级故障阀值", "三级故障阀值", "加热控制参数", "充电控制参数", "电池信息"] string[] ["从板信息", "一级故障阀值", "二级故障阀值", "三级故障阀值", "均衡参数"]] -> w4191
              tunnel: [0.0 ("从板号") w4323] -> w4195
              tunnel: [w4308 _] -> w4193
              tunnel: [_ w4324] -> w4192
              frame "主板", Default {
                n3166 = stacked-sequence {
                  tunnel: [_ w4322] -> w4308
                  frame #0 {
                    n3167 = control-ref of="电池信息"() -> (w4314:refnum<vi>)
                    n3168 = control-ref of="高压参数"() -> (w4313:refnum<vi>)
                    n3169 = control-ref of="一级故障"() -> (w4316:refnum<vi>)
                    n3170 = control-ref of="一级故障 2"() -> (w4318:refnum<vi>)
                    n3171 = control-ref of="一级故障 3"() -> (w4319:refnum<vi>)
                    n3172 = control-ref of="加热控制参数"() -> (w4320:refnum<vi>)
                    n3173 = control-ref of="充电控制参数"() -> (w4321:refnum<vi>)
                    n3174 = control-ref of="项目信息"() -> (w4317:refnum<vi>)
                    n3175 = control-ref of="项目信息2"() -> (w4315:refnum<vi>)
                    n3176 = local read "主板数据"() -> (w4312:T4)
                    n3177 = Bundle(cluster=w4312, "项目信息"=w4317, "一级故障 4"=w4315, "一级故障"=w4316, "一级故障 2"=w4318, "一级故障 3"=w4319, "加热控制参数"=w4320, "充电控制参数"=w4321, "高压参数"=w4313, "电池信息"=w4314) -> (w4311:T4)
                    n3178 = local write "主板数据"(w4311) -> ()
                  }
                  frame #1 {
                    n3179 = control-ref of="主板数据"() -> (w4322:refnum<vi>)
                  }
                }
              }
              frame "从板" {
                (unwired) "均衡参数"
                n3180 = stacked-sequence {
                  tunnel: [_ w4336] -> w4324
                  frame #0 {
                    n3181 = control-ref of="从板号"() -> (w4330:refnum<vi>)
                    n3182 = control-ref of="项目信息 2"() -> (w4331:refnum<vi>)
                    n3183 = control-ref of="均衡参数"() -> (w4328:refnum<vi>)
                    n3184 = control-ref of="加热控制参数"() -> (w4332:refnum<vi>)
                    n3185 = control-ref of="一级故障(从板)"() -> (w4333:refnum<vi>)
                    n3186 = control-ref of="二级故障(从板)"() -> (w4334:refnum<vi>)
                    n3187 = control-ref of="三级故障(从板)"() -> (w4335:refnum<vi>)
                    n3188 = control-ref of="电池组信息"() -> (w4329:refnum<vi>)
                    n3189 = local read "从板信息"() -> (w4327:T2)
                    n3190 = Bundle(cluster=w4327, "从板号"=w4330, "项目信息 2"=w4331, "加热控制参数"=w4332, "一级故障(从板)"=w4333, "二级故障(从板)"=w4334, "三级故障(从板)"=w4335, "电池组信息(从板)"=w4329, "均衡参数"=w4328) -> (w4326:T2)
                    n3191 = local write "从板信息"(w4326) -> ()
                  }
                  frame #1 {
                    n3192 = control-ref of="从板信息"() -> (w4336:refnum<vi>)
                  }
                }
                n3193 = local read "从板号"() -> (w4323:u8)
              }
            }
            n3194 = Array Size(array=w4191) -> (size(s)=w4190:i32)
            n3195 = while {
              tunnel: w4191 -> [w4203] mode=indexing
              tunnel: w4194 -> [w4207]
              tunnel: w4195 -> [w4210]
              tunnel: w4193 -> [w4209]
              tunnel: w4192 -> [w4208]
              tunnel: w4190 -> [w4201]
              tunnel: [w4197] -> w4189
              i -> [w4202]
              stop <- w4198 stop-if-true
              n3196 = Increment(x=w4202) -> (x+1=w4200:i32)
              n3197 = local read "从板个数"() -> (w4215:dbl)
              n3198 = local read "快换"() -> (w4206:bool)
              n3199 = Less Or Equal?(x=w4201, y=w4200) -> (x <= y?=w4197:bool)
              n3200 = call "输入数据解析.vi"("单个参数补充"=w4215, "从板号"=w4210, "主板引用"=w4209, "从板引用"=w4208, "主板选项"=w4203, "枚举"=w4207, "快换"=w4206) -> ("输出数组"=w4214:dbl[][], "数组长度"=w4213:dbl[], "循环次数"=w4205:i32, "命令"=w4212:u32, "名称"=w4204:string[], "命令序号"=w4211:u32[])  [unwired: 2 in, 1 out]
              n3201 = case shown="\"主板\", 默认" w4207 {
                tunnel: w4202 -> [w4217 w4231]
                frame "主板", Default {
                  n3202 = case shown="6" w4217 {
                    tunnel: [T8."项目信息" ("主从板") T8."一级故障阀值" ("主从板") T8."二级故障阀值" ("主从板") T8."三级故障阀值" ("主从板") T8."控制参数" ("主从板") T8."电池信息" ("主从板")] -> w4216
                    frame 0, Default {
                      n3203 = local write "1"(TRUE ("1")) -> ()
                    }
                    frame 1 {
                      n3204 = local write "1 2"(TRUE ("1 2")) -> ()
                    }
                    frame 2 {
                      n3205 = local write "1 3"(TRUE ("1 3")) -> ()
                    }
                    frame 3 {
                      n3206 = local write "1 4"(TRUE ("1 4")) -> ()
                    }
                    frame 4, 5 {
                      n3207 = local write "1 5"(TRUE ("1 5")) -> ()
                    }
                    frame 6 {
                      n3208 = local write "1 11"(TRUE ("1 11")) -> ()
                    }
                  }
                  n3209 = local write "主板2"(w4216) -> ()
                }
                frame "从板" {
                  n3210 = case shown="1" w4231 {
                    tunnel: [T19."从板信息" ("等级 2") T19."从板信息" ("等级 2") T19."一级故障阀值" ("等级 2") T19."二级故障阀值" ("等级 2") T19."三级故障阀值" ("等级 2") T19."快换参数" ("等级 2") T14."均衡参数" ("等级 2")] -> w4230
                    frame 99, Default {
                      n3211 = local write "1 6"(TRUE ("1 6")) -> ()
                    }
                    frame 0 {
                      n3212 = local write "1 6"(TRUE ("1 6")) -> ()
                    }
                    frame 1 {
                      n3213 = local write "1 7"(TRUE ("1 7")) -> ()
                    }
                    frame 2 {
                      n3214 = local write "1 8"(TRUE ("1 8")) -> ()
                    }
                    frame 3 {
                      n3215 = local write "1 9"(TRUE ("1 9")) -> ()
                    }
                    frame 4 {
                      n3216 = local write "1 10"(TRUE ("1 10")) -> ()
                    }
                    frame 5 {
                      n3217 = local write "1 12"(TRUE ("1 10")) -> ()
                    }
                  }
                  n3218 = local write "等级 2"(w4230) -> ()
                }
              }
              n3219 = for {
                N: w4205 -> [w4248]
                tunnel: w4214 -> [w4258]
                tunnel: w4213 -> [w4257]
                tunnel: w4212 -> [w4256]
                tunnel: w4211 -> [w4254]
                tunnel: w4210 -> [w4255]
                tunnel: w4204 -> [w4251]
                tunnel: w4197 -> [w4246]
                i -> [w4247]
                n3220 = Index Array(array=w4258, index (row)=w4247) -> (element=w4253:dbl[])  [unwired: 1 in]
                n3221 = Index Array(array=w4257, index=w4247) -> (element=w4252:dbl)
                n3222 = Index Array(array=w4251, index=w4247) -> (element=w4249:string)
                n3223 = Index Array(array=w4254, index=w4247) -> (element=w4250:u32)
                n3224 = stacked-sequence {
                  seq-local: [_ _ _ w4281 _ _] -> [_ _ _ _ w4290 _]
                  tunnel: w4253 -> [_ _ w4269 _ _ _]
                  tunnel: w4252 -> [_ _ w4268 _ _ _]
                  tunnel: w4256 -> [_ _ w4263 _ _ _]
                  tunnel: w4255 -> [_ _ w4266 _ _ _]
                  tunnel: w4250 -> [_ _ w4264 _ _ _]
                  tunnel: w4249 -> [_ _ w4262 _ w4289 _]
                  tunnel: w4248 -> [_ _ _ _ _ w4302]
                  tunnel: w4247 -> [_ _ _ _ _ w4301]
                  tunnel: w4246 -> [_ _ _ _ _ w4299]
                  frame #0 {
                    w4260 = FALSE ("流控帧")
                    w4259 = TRUE ("流控帧 2")
                    n3225 = call <vilib>:"Set Busy.vi"("disable click? (T)"=w4260) -> ()  [unwired: 3 in, 8 out]
                    n3226 = global write "EV05全局变量1.vi" "读取超时"(w4260) -> ()
                    n3227 = global write "EV05全局变量1.vi" "流控帧"(w4260) -> ()
                    n3228 = local write "消除"(w4259) -> ()
                    n3229 = local write "控制1"(w4259) -> ()
                    n3230 = global write "EV05全局变量1.vi" "流控帧 2"(w4259) -> ()
                    n3231 = local write "写?"(w4259) -> ()
                  }
                  frame #1 {
                    n3232 = Wait Until Next ms Multiple(millisecond multiple=u32 50 ("毫秒倍数")) -> ()  [unwired: 1 out]
                  }
                  frame #2 {
                    n3233 = global write "全局 1.vi" "名称"(w4262) -> ()
                    n3234 = local write "命令序号"(w4264) -> ()
                    n3235 = local write "命令"(w4263) -> ()
                    n3236 = local read "设备索引号"() -> (w4271:u16)
                    n3237 = local read "CAN卡类型"() -> (w4272:u32)
                    n3238 = Increment(x=w4268) -> (x+1=w4265:dbl)
                    n3239 = local read "CAN端口"() -> (w4270:u16)
                    n3240 = Reshape Array(w4269, w4265) -> (w4267:dbl[])
                    n3241 = stacked-sequence {
                      tunnel: w4272 -> [_ w4280]
                      tunnel: w4271 -> [_ w4279]
                      tunnel: w4270 -> [_ w4278]
                      tunnel: w4267 -> [_ w4277]
                      tunnel: w4266 -> [_ w4276]
                      tunnel: w4264 -> [_ w4275]
                      tunnel: w4263 -> [_ w4274]
                      frame #0 {
                      }
                      frame #1 {
                        n3242 = call "多帧发送机制(EV05).vi"("can卡类型"=w4280, "设备索引号"=w4279, "CAN端口"=w4278, "命令"=w4274, "板号"=w4276, "命令序号"=w4275, "输入数据"=w4277) -> ("错误输出"=w4273:errorcluster)  [unwired: 1 in, 11 out]
                        n3243 = call <vilib>:"Clear Errors.vi"("error in (no error)"=w4273) -> ()  [unwired: 6 in, 1 out]
                      }
                    }
                  }
                  frame #3 {
                    n3244 = while {
                      tunnel: [w4283] -> w4281
                      i -> [w4288]
                      stop <- w4285 stop-if-true
                      n3245 = local read "强制终止读写标记"() -> (w4282:bool)
                      n3246 = global read "EV05全局变量1.vi" "读取超时"() -> (w4283:bool)
                      n3247 = Greater Or Equal?(x=w4288, y=30) -> (x >= y?=w4286:bool)
                      n3248 = Wait Until Next ms Multiple(millisecond multiple=u32 100 ("毫秒倍数")) -> ()  [unwired: 1 out]
                      n3249 = Compound Arithmetic op=OR(w4282, w4283, w4286) -> (w4285:bool)
                    }
                  }
                  frame #4 {
                    n3250 = call <vilib>:"Unset Busy.vi"() -> ()  [unwired: 2 in, 10 out]
                    n3251 = case shown="假" w4290 {
                      tunnel: w4289 -> [w4291 _]
                      frame False {
                        n3252 = control-ref of="结果"() -> (w4295:refnum<vi>)
                        n3253 = Concatenate Strings(w4291, "       写入失败" ("字符串")) -> (w4294:string)
                        n3254 = Build Array(w4294) -> (w4293:string[])
                        n3255 = call "表格编辑.vi"("新元素/子数组"=w4293, "活动单元格:单元格背景色"=u32 16740749, "MCListbox引用句柄"=w4295) -> ()  [unwired: 9 out]
                      }
                      frame True {
                      }
                    }
                  }
                  frame #5 {
                    n3256 = Increment(x=w4301) -> (x+1=w4297:i32)
                    n3257 = Equal?(x=w4302, y=w4297) -> (x = y?=w4300:bool)
                    n3258 = And(x=w4299, y=w4300) -> (x .and. y?=w4298:bool)
                    n3259 = case shown="真" w4298 {
                      frame False {
                      }
                      frame True {
                        n3260 = control-ref of="结果"() -> (w4306:refnum<vi>)
                        n3261 = Concatenate Strings("写入完成" ("字符串")) -> (w4305:string)
                        n3262 = Build Array(w4305) -> (w4304:string[])
                        n3263 = call "表格编辑.vi"("新元素/子数组"=w4304, "活动单元格:单元格背景色"=u32 21937, "MCListbox引用句柄"=w4306) -> ()  [unwired: 9 out]
                      }
                    }
                  }
                }
              }
              n3264 = local read "强制终止读写标记"() -> (w4199:bool)
              n3265 = Or(x=w4197, y=w4199) -> (x .or. y?=w4198:bool)
            }
            n3266 = stacked-sequence {
              tunnel: w4189 -> [_]
              frame #0 {
                n3267 = call <vilib>:"Unset Busy.vi"() -> ()  [unwired: 2 in, 10 out]
                n3268 = local write "强制终止读写标记"(FALSE ("强制停止")) -> ()
              }
            }
          }
          frame "单个读取" {
            n3269 = stacked-sequence {
              tunnel: [w4339] -> w4337
              frame #0 {
                n3270 = local read "主从选择"() -> (w4340:enum32{"主板", "从板"})
                n3271 = case shown="\"主板\", 默认" w4340 {
                  tunnel: [w4353 w4436] -> w4342
                  tunnel: [w4352 w4437] -> w4347
                  tunnel: [0 ("从板号") w4433] -> w4346
                  tunnel: [0 ("板号") u8 0 ("板号")] -> w4345
                  tunnel: [w4348 w4432] -> w4343
                  frame "主板", Default {
                    n3272 = local read "主板选项"() -> (w4349:string)
                    n3273 = case shown="\"二维码\"" w4349 {
                      tunnel: [_ u8[] [1, 2, 3, 4, 5, 6, 13, 8, 7, 9, 10, 11, 12] u8[] [1] u8[] [1] u8[] [1] u8[] [2] u8[] [3] u8[] [4] u8[] [5] u8[] [6] u8[] [13] u8[] [7] u8[] [8] u8[] [9] u8[] [10] u8[] [14] u8[] [11] u8[] [12] u8[] [2] u8[] [3] u8[] [1] u8[] [2] u8[] [1] u8[] [2] u8[] [3] u8[] [4] u8[] [1, 2, 3, 4]] -> w4353
